vi "LabVIEW_MQTT_Toolkit_V2.vi"() -> ()   [LabVIEW 2021] (continued)
                n724 = Open/Create/Replace File(file path (use dialog)=w1674, operation (0:open)=T11."open or create") -> (refnum out=w1667:refnum<file>, error out=w1665:errorcluster)  [unwired: 4 in, 1 out]
                n725 = Write to Text File(file (use dialog)=w1667, text=w1668, error in=w1665) -> (refnum out=w1666:refnum<file>, error out=w1664:errorcluster)  [unwired: 1 in, 1 out]
                n726 = Close File(refnum=w1666, error in=w1664) -> (path=w1654:path)  [unwired: 1 out]
              }
              frame 19 {
                w1723 = T14 2 items=["User Home"=0, "User Desktop"=1, "User Documents"=2, "User Application Data"=3, "User Preferences"=4, "User Temporary"=5, "Public Documents"=6, "Public Application Data"=7, "Public Preferences"=8, "Public Cache"=13, "System Core Libraries"=9, "System Installed Libraries"=10, "Application Files"=11, "Boot Volume Root"=12] ("system directory type")
                n727 = Search and Replace String(replace all?=TRUE ("replace all? (F)"), input string=w1718, search string="/") -> (result string=w1739:string)  [unwired: 5 in, 3 out]
                n728 = Concatenate Strings(w1716, "TimeStamp;MeasureCh_Z(g);Ch_X(g);INC_Y(Deg)", "\n") -> (w1732:string)
                n729 = Concatenate Strings(w1739, "_" ("string"), "streaming.csv") -> (w1740:string)
                n730 = call <vilib>:"Get System Directory.vi"("system directory type"=w1723) -> ("system directory"=w1733:path)  [unwired: 10 in]
                n731 = Decimate 1D Array(w1756) -> (w1752:dbl[], w1751:dbl[], w1754:dbl[])
                n732 = for {
                  tunnel: [w1784] -> w1753 mode=indexing
                  tunnel: w1755 -> [w1778] mode=indexing
                  tunnel: w1752 -> [w1777] mode=indexing
                  tunnel: w1751 -> [w1776] mode=indexing
                  tunnel: w1754 -> [w1775] mode=indexing
                  tunnel: [w1777] -> w1750 mode=indexing
                  tunnel: [w1776] -> w1749 mode=indexing
                  tunnel: [w1775] -> w1748 mode=indexing
                  tunnel: w1747 -> [w1770]
                  tunnel: w1746 -> [w1769]
                  tunnel: w1745 -> [w1768] mode=indexing
                  tunnel: w1744 -> [w1767]
                  tunnel: [w1761] -> w1743
                  tunnel: [w1761] -> w1742
                  tunnel: [w1761] -> w1741
                  n733 = Join Numbers(hi=w1770, lo=w1769) -> ((hi.lo)=w1772:u32)
                  n734 = To Double Precision Float(number=w1768) -> (double precision float=w1773:dbl)
                  n735 = Number To Decimal String(number=w1778) -> (decimal integer string=w1783:string)  [unwired: 1 in]
                  n736 = Number To Fractional String(number=w1777, precision (6)=i16 3 ("width (-)")) -> (F-format string=w1785:string)  [unwired: 2 in]
                  n737 = Number To Fractional String(number=w1776, precision (6)=i16 3 ("width (-)")) -> (F-format string=w1781:string)  [unwired: 2 in]
                  n738 = Number To Fractional String(number=w1775, precision (6)=i16 3 ("width (-)")) -> (F-format string=w1779:string)  [unwired: 2 in]
                  n739 = Divide(x=w1773, y=w1767) -> (x/y=w1774:dbl)
                  n740 = To Unsigned Quad Integer(1:w1772) -> (0:w1771:u64)
                  n741 = Build Array(w1783, w1785, w1781, w1779) -> (w1784:string[])
                  n742 = call "Unix Time to Timestamp.vi"("Fractional Second"=w1774, "Unix Time (s)"=w1771) -> ("Timestamp"=w1762:timestamp)  [unwired: 8 in, 1 out]
                  n743 = Format Date/Time String(seconds (now)=w1762, UTC format=TRUE) -> (date/time string=w1763:string)  [unwired: 1 in]
                  n744 = Scan From String(format string="%<%x %H:%M:%S%3u>T", input string=w1763) -> (output 1=w1764:timestamp)  [unwired: 3 in, 3 out]
                  n745 = To Double Precision Float(number=w1764) -> (double precision float=w1761:dbl)
                }
                n746 = Build Path(base path=w1733, name or relative path="Logfile") -> (appended path=w1734:path)
                n747 = call <vilib>:"Check if File or Folder Exists.vi"("path"=w1734) -> ("file or folder exists?"=w1735:bool, "dup path"=w1736:path)  [unwired: 8 in, 1 out]
                n748 = case shown="False" w1735 {
                  tunnel: w1736 -> [w1759 w1760]
                  tunnel: [w1758 w1760] -> w1737
                  frame False {
                    n749 = Create Folder(path (use dialog)=w1759) -> (created path=w1758:path)  [unwired: 2 in, 2 out]
                  }
                  frame True {
                  }
                }
                n750 = Build Path(base path=w1737, name or relative path=w1740) -> (appended path=w1738:path)
                n751 = Open/Create/Replace File(file path (use dialog)=w1738, operation (0:open)=T11."open or create") -> (refnum out=w1731:refnum<file>, error out=w1729:errorcluster)  [unwired: 4 in, 1 out]
                n752 = Write to Text File(file (use dialog)=w1731, text=w1732, error in=w1729) -> (refnum out=w1730:refnum<file>, error out=w1728:errorcluster)  [unwired: 1 in, 1 out]
                n753 = Close File(refnum=w1730, error in=w1728) -> (path=w1717:path)  [unwired: 1 out]
              }
              frame 20 {
                w1794 = T14 2 items=["User Home"=0, "User Desktop"=1, "User Documents"=2, "User Application Data"=3, "User Preferences"=4, "User Temporary"=5, "Public Documents"=6, "Public Application Data"=7, "Public Preferences"=8, "Public Cache"=13, "System Core Libraries"=9, "System Installed Libraries"=10, "Application Files"=11, "Boot Volume Root"=12] ("system directory type")
                n754 = Decimate 1D Array(w1823) -> (w1819:dbl[], w1821:dbl[])
                n755 = Search and Replace String(replace all?=TRUE ("replace all? (F)"), input string=w1788, search string="/") -> (result string=w1810:string)  [unwired: 5 in, 3 out]
                n756 = for {
                  tunnel: [w1848] -> w1820 mode=indexing
                  tunnel: w1822 -> [w1844] mode=indexing
                  tunnel: w1819 -> [w1843] mode=indexing
                  tunnel: w1821 -> [w1842] mode=indexing
                  tunnel: [w1843] -> w1818 mode=indexing
                  tunnel: [w1842] -> w1817 mode=indexing
                  tunnel: w1816 -> [w1837]
                  tunnel: w1815 -> [w1836]
                  tunnel: w1814 -> [w1835] mode=indexing
                  tunnel: w1813 -> [w1834]
                  tunnel: [w1828] -> w1812
                  n757 = Join Numbers(hi=w1837, lo=w1836) -> ((hi.lo)=w1839:u32)
                  n758 = To Double Precision Float(number=w1835) -> (double precision float=w1840:dbl)
                  n759 = Number To Decimal String(number=w1844) -> (decimal integer string=w1847:string)  [unwired: 1 in]
                  n760 = Number To Fractional String(number=w1843, precision (6)=i16 3 ("width (-)")) -> (F-format string=w1849:string)  [unwired: 2 in]
                  n761 = Number To Fractional String(number=w1842, precision (6)=i16 3 ("width (-)")) -> (F-format string=w1845:string)  [unwired: 2 in]
                  n762 = Divide(x=w1840, y=w1834) -> (x/y=w1841:dbl)
                  n763 = Build Array(w1847, w1849, w1845) -> (w1848:string[])
                  n764 = To Unsigned Quad Integer(1:w1839) -> (0:w1838:u64)
                  n765 = call "Unix Time to Timestamp.vi"("Fractional Second"=w1841, "Unix Time (s)"=w1838) -> ("Timestamp"=w1829:timestamp)  [unwired: 8 in, 1 out]
                  n766 = Format Date/Time String(seconds (now)=w1829, UTC format=TRUE) -> (date/time string=w1830:string)  [unwired: 1 in]
                  n767 = Scan From String(format string="%<%x %H:%M:%S%3u>T", input string=w1830) -> (output 1=w1831:timestamp)  [unwired: 3 in, 3 out]
                  n768 = To Double Precision Float(number=w1831) -> (double precision float=w1828:dbl)
                }
                n769 = Concatenate Strings(w1787, "TimeStamp;MeasureCh_Y(g);INC_Y(Deg)", "\n") -> (w1803:string)
                n770 = Concatenate Strings(w1810, "_" ("string"), "streaming.csv") -> (w1811:string)
                n771 = call <vilib>:"Get System Directory.vi"("system directory type"=w1794) -> ("system directory"=w1804:path)  [unwired: 10 in]
                n772 = Build Path(base path=w1804, name or relative path="Logfile") -> (appended path=w1805:path)
                n773 = call <vilib>:"Check if File or Folder Exists.vi"("path"=w1805) -> ("file or folder exists?"=w1806:bool, "dup path"=w1807:path)  [unwired: 8 in, 1 out]
                n774 = case shown="False" w1806 {
                  tunnel: w1807 -> [w1826 w1827]
                  tunnel: [w1825 w1827] -> w1808
                  frame False {
                    n775 = Create Folder(path (use dialog)=w1826) -> (created path=w1825:path)  [unwired: 2 in, 2 out]
                  }
                  frame True {
                  }
                }
                n776 = Build Path(base path=w1808, name or relative path=w1811) -> (appended path=w1809:path)
                n777 = Open/Create/Replace File(file path (use dialog)=w1809, operation (0:open)=T11."open or create") -> (refnum out=w1802:refnum<file>, error out=w1800:errorcluster)  [unwired: 4 in, 1 out]
                n778 = Write to Text File(file (use dialog)=w1802, text=w1803, error in=w1800) -> (refnum out=w1801:refnum<file>, error out=w1799:errorcluster)  [unwired: 1 in, 1 out]
                n779 = Close File(refnum=w1801, error in=w1799) -> (path=w1789:path)  [unwired: 1 out]
              }
              frame 21 {
                w1858 = T14 2 items=["User Home"=0, "User Desktop"=1, "User Documents"=2, "User Application Data"=3, "User Preferences"=4, "User Temporary"=5, "Public Documents"=6, "Public Application Data"=7, "Public Preferences"=8, "Public Cache"=13, "System Core Libraries"=9, "System Installed Libraries"=10, "Application Files"=11, "Boot Volume Root"=12] ("system directory type")
                n780 = Search and Replace String(replace all?=TRUE ("replace all? (F)"), input string=w1853, search string="/") -> (result string=w1874:string)  [unwired: 5 in, 3 out]
                n781 = Concatenate Strings(w1851, "TimeStamp;MeasureCh_Z(g);Ch_Y(g);INC_Y(Deg)", "\n") -> (w1867:string)
                n782 = Concatenate Strings(w1874, "_" ("string"), "streaming.csv") -> (w1875:string)
                n783 = call <vilib>:"Get System Directory.vi"("system directory type"=w1858) -> ("system directory"=w1868:path)  [unwired: 10 in]
                n784 = Decimate 1D Array(w1891) -> (w1887:dbl[], w1886:dbl[], w1889:dbl[])
                n785 = for {
                  tunnel: [w1919] -> w1888 mode=indexing
                  tunnel: w1890 -> [w1913] mode=indexing
                  tunnel: w1887 -> [w1912] mode=indexing
                  tunnel: w1886 -> [w1911] mode=indexing
                  tunnel: w1889 -> [w1910] mode=indexing
                  tunnel: [w1912] -> w1885 mode=indexing
                  tunnel: [w1911] -> w1884 mode=indexing
                  tunnel: [w1910] -> w1883 mode=indexing
                  tunnel: w1882 -> [w1905]
                  tunnel: w1881 -> [w1904]
                  tunnel: w1880 -> [w1903] mode=indexing
                  tunnel: w1879 -> [w1902]
                  tunnel: [w1896] -> w1878
                  tunnel: [w1896] -> w1877
                  tunnel: [w1896] -> w1876
                  n786 = Join Numbers(hi=w1905, lo=w1904) -> ((hi.lo)=w1907:u32)
                  n787 = To Double Precision Float(number=w1903) -> (double precision float=w1908:dbl)
                  n788 = Number To Decimal String(number=w1913) -> (decimal integer string=w1918:string)  [unwired: 1 in]
                  n789 = Number To Fractional String(number=w1912, precision (6)=i16 3 ("width (-)")) -> (F-format string=w1920:string)  [unwired: 2 in]
                  n790 = Number To Fractional String(number=w1911, precision (6)=i16 3 ("width (-)")) -> (F-format string=w1916:string)  [unwired: 2 in]
                  n791 = Number To Fractional String(number=w1910, precision (6)=i16 3 ("width (-)")) -> (F-format string=w1914:string)  [unwired: 2 in]
                  n792 = Divide(x=w1908, y=w1902) -> (x/y=w1909:dbl)
                  n793 = To Unsigned Quad Integer(1:w1907) -> (0:w1906:u64)
                  n794 = Build Array(w1918, w1920, w1916, w1914) -> (w1919:string[])
                  n795 = call "Unix Time to Timestamp.vi"("Fractional Second"=w1909, "Unix Time (s)"=w1906) -> ("Timestamp"=w1897:timestamp)  [unwired: 8 in, 1 out]
                  n796 = Format Date/Time String(seconds (now)=w1897, UTC format=TRUE) -> (date/time string=w1901:string)  [unwired: 1 in]
                  n797 = Scan From String(format string="%<%x %H:%M:%S%3u>T", input string=w1901) -> (output 1=w1900:timestamp)  [unwired: 3 in, 3 out]
                  n798 = To Double Precision Float(number=w1900) -> (double precision float=w1896:dbl)
                }
                n799 = Build Path(base path=w1868, name or relative path="Logfile") -> (appended path=w1869:path)
                n800 = call <vilib>:"Check if File or Folder Exists.vi"("path"=w1869) -> ("file or folder exists?"=w1870:bool, "dup path"=w1871:path)  [unwired: 8 in, 1 out]
                n801 = case shown="False" w1870 {
                  tunnel: w1871 -> [w1894 w1895]
                  tunnel: [w1893 w1895] -> w1872
                  frame False {
                    n802 = Create Folder(path (use dialog)=w1894) -> (created path=w1893:path)  [unwired: 2 in, 2 out]
                  }
                  frame True {
                  }
                }
                n803 = Build Path(base path=w1872, name or relative path=w1875) -> (appended path=w1873:path)
                n804 = Open/Create/Replace File(file path (use dialog)=w1873, operation (0:open)=T11."open or create") -> (refnum out=w1866:refnum<file>, error out=w1864:errorcluster)  [unwired: 4 in, 1 out]
                n805 = Write to Text File(file (use dialog)=w1866, text=w1867, error in=w1864) -> (refnum out=w1865:refnum<file>, error out=w1863:errorcluster)  [unwired: 1 in, 1 out]
                n806 = Close File(refnum=w1865, error in=w1863) -> (path=w1852:path)  [unwired: 1 out]
              }
              frame 22 {
                w1929 = T14 2 items=["User Home"=0, "User Desktop"=1, "User Documents"=2, "User Application Data"=3, "User Preferences"=4, "User Temporary"=5, "Public Documents"=6, "Public Application Data"=7, "Public Preferences"=8, "Public Cache"=13, "System Core Libraries"=9, "System Installed Libraries"=10, "Application Files"=11, "Boot Volume Root"=12] ("system directory type")
                n807 = Search and Replace String(replace all?=TRUE ("replace all? (F)"), input string=w1924, search string="/") -> (result string=w1945:string)  [unwired: 5 in, 3 out]
                n808 = Concatenate Strings(w1922, "TimeStamp;MeasureCh_X(g);Ch_Y(g);INC_X(Deg)", "\n") -> (w1938:string)
                n809 = Concatenate Strings(w1945, "_" ("string"), "streaming.csv") -> (w1946:string)
                n810 = call <vilib>:"Get System Directory.vi"("system directory type"=w1929) -> ("system directory"=w1939:path)  [unwired: 10 in]
                n811 = Decimate 1D Array(w1962) -> (w1958:dbl[], w1957:dbl[], w1961:dbl[])
                n812 = for {
                  tunnel: [w1990] -> w1959 mode=indexing
                  tunnel: w1960 -> [w1984] mode=indexing
                  tunnel: w1958 -> [w1983] mode=indexing
                  tunnel: w1957 -> [w1982] mode=indexing
                  tunnel: w1961 -> [w1981] mode=indexing
                  tunnel: [w1983] -> w1956 mode=indexing
                  tunnel: [w1982] -> w1955 mode=indexing
                  tunnel: [w1981] -> w1954 mode=indexing
                  tunnel: w1953 -> [w1976]
                  tunnel: w1952 -> [w1975]
                  tunnel: w1951 -> [w1974] mode=indexing
                  tunnel: w1950 -> [w1973]
                  tunnel: [w1967] -> w1949
                  tunnel: [w1967] -> w1948
                  tunnel: [w1967] -> w1947
                  n813 = Join Numbers(hi=w1976, lo=w1975) -> ((hi.lo)=w1978:u32)
                  n814 = To Double Precision Float(number=w1974) -> (double precision float=w1979:dbl)
                  n815 = Number To Decimal String(number=w1984) -> (decimal integer string=w1989:string)  [unwired: 1 in]
                  n816 = Number To Fractional String(number=w1983, precision (6)=i16 3 ("width (-)")) -> (F-format string=w1991:string)  [unwired: 2 in]
                  n817 = Number To Fractional String(number=w1982, precision (6)=i16 3 ("width (-)")) -> (F-format string=w1987:string)  [unwired: 2 in]
                  n818 = Number To Fractional String(number=w1981, precision (6)=i16 3 ("width (-)")) -> (F-format string=w1985:string)  [unwired: 2 in]
                  n819 = Divide(x=w1979, y=w1973) -> (x/y=w1980:dbl)
                  n820 = To Unsigned Quad Integer(1:w1978) -> (0:w1977:u64)
                  n821 = Build Array(w1989, w1991, w1987, w1985) -> (w1990:string[])
                  n822 = call "Unix Time to Timestamp.vi"("Fractional Second"=w1980, "Unix Time (s)"=w1977) -> ("Timestamp"=w1968:timestamp)  [unwired: 8 in, 1 out]
                  n823 = Format Date/Time String(seconds (now)=w1968, UTC format=TRUE) -> (date/time string=w1969:string)  [unwired: 1 in]
                  n824 = Scan From String(format string="%<%x %H:%M:%S%3u>T", input string=w1969) -> (output 1=w1970:timestamp)  [unwired: 3 in, 3 out]
                  n825 = To Double Precision Float(number=w1970) -> (double precision float=w1967:dbl)
                }
                n826 = Build Path(base path=w1939, name or relative path="Logfile") -> (appended path=w1940:path)
                n827 = call <vilib>:"Check if File or Folder Exists.vi"("path"=w1940) -> ("file or folder exists?"=w1941:bool, "dup path"=w1942:path)  [unwired: 8 in, 1 out]
                n828 = case shown="False" w1941 {
                  tunnel: w1942 -> [w1965 w1966]
                  tunnel: [w1964 w1966] -> w1943
                  frame False {
                    n829 = Create Folder(path (use dialog)=w1965) -> (created path=w1964:path)  [unwired: 2 in, 2 out]
                  }
                  frame True {
                  }
                }
                n830 = Build Path(base path=w1943, name or relative path=w1946) -> (appended path=w1944:path)
                n831 = Open/Create/Replace File(file path (use dialog)=w1944, operation (0:open)=T11."open or create") -> (refnum out=w1937:refnum<file>, error out=w1935:errorcluster)  [unwired: 4 in, 1 out]
                n832 = Write to Text File(file (use dialog)=w1937, text=w1938, error in=w1935) -> (refnum out=w1936:refnum<file>, error out=w1934:errorcluster)  [unwired: 1 in, 1 out]
                n833 = Close File(refnum=w1936, error in=w1934) -> (path=w1923:path)  [unwired: 1 out]
              }
              frame 23 {
                w2000 = T14 2 items=["User Home"=0, "User Desktop"=1, "User Documents"=2, "User Application Data"=3, "User Preferences"=4, "User Temporary"=5, "Public Documents"=6, "Public Application Data"=7, "Public Preferences"=8, "Public Cache"=13, "System Core Libraries"=9, "System Installed Libraries"=10, "Application Files"=11, "Boot Volume Root"=12] ("system directory type")
                n834 = Search and Replace String(replace all?=TRUE ("replace all? (F)"), input string=w1994, search string="/") -> (result string=w2016:string)  [unwired: 5 in, 3 out]
                n835 = Concatenate Strings(w1993, "TimeStamp;MeasureCh_Z(g);Ch_X(g);Ch_Y(g);INC_Y(Deg)", "\n") -> (w2009:string)
                n836 = Concatenate Strings(w2016, "_" ("string"), "streaming.csv") -> (w2017:string)
                n837 = call <vilib>:"Get System Directory.vi"("system directory type"=w2000) -> ("system directory"=w2010:path)  [unwired: 10 in]
                n838 = Decimate 1D Array(w2033) -> (w2032:dbl[], w2031:dbl[], w2030:dbl[], w2027:dbl[])
                n839 = for {
                  tunnel: [w2063] -> w2028 mode=indexing
                  tunnel: w2029 -> [w2057] mode=indexing
                  tunnel: w2032 -> [w2055] mode=indexing
                  tunnel: w2031 -> [w2054] mode=indexing
                  tunnel: w2030 -> [w2053] mode=indexing
                  tunnel: w2027 -> [w2052] mode=indexing
                  tunnel: [w2055] -> w2026 mode=indexing
                  tunnel: [w2054] -> w2025 mode=indexing
                  tunnel: [w2053] -> w2024 mode=indexing
                  tunnel: [w2052] -> w2023 mode=indexing
                  tunnel: w2022 -> [w2047]
                  tunnel: w2021 -> [w2046]
                  tunnel: w2020 -> [w2045] mode=indexing
                  tunnel: w2019 -> [w2044]
                  tunnel: [w2038] -> w2018
                  n840 = Number To Fractional String(number=w2052, precision (6)=i16 3 ("width (-)")) -> ()  [unwired: 2 in, 1 out]
                  n841 = Join Numbers(hi=w2047, lo=w2046) -> ((hi.lo)=w2049:u32)
                  n842 = To Double Precision Float(number=w2045) -> (double precision float=w2050:dbl)
                  n843 = Number To Decimal String(number=w2057) -> (decimal integer string=w2062:string)  [unwired: 1 in]
                  n844 = Number To Fractional String(number=w2055, precision (6)=i16 3 ("width (-)")) -> (F-format string=w2064:string)  [unwired: 2 in]
                  n845 = Number To Fractional String(number=w2054, precision (6)=i16 3 ("width (-)")) -> (F-format string=w2060:string)  [unwired: 2 in]
                  n846 = Number To Fractional String(number=w2053, precision (6)=i16 3 ("width (-)")) -> (F-format string=w2058:string)  [unwired: 2 in]
                  n847 = Divide(x=w2050, y=w2044) -> (x/y=w2051:dbl)
                  n848 = To Unsigned Quad Integer(1:w2049) -> (0:w2048:u64)
                  n849 = Build Array(w2062, w2064, w2060, w2058) -> (w2063:string[])
                  n850 = call "Unix Time to Timestamp.vi"("Fractional Second"=w2051, "Unix Time (s)"=w2048) -> ("Timestamp"=w2039:timestamp)  [unwired: 8 in, 1 out]
                  n851 = Format Date/Time String(seconds (now)=w2039, UTC format=TRUE) -> (date/time string=w2040:string)  [unwired: 1 in]
                  n852 = Scan From String(format string="%<%x %H:%M:%S%3u>T", input string=w2040) -> (output 1=w2041:timestamp)  [unwired: 3 in, 3 out]
                  n853 = To Double Precision Float(number=w2041) -> (double precision float=w2038:dbl)
                }
                n854 = Build Path(base path=w2010, name or relative path="Logfile") -> (appended path=w2011:path)
                n855 = call <vilib>:"Check if File or Folder Exists.vi"("path"=w2011) -> ("file or folder exists?"=w2012:bool, "dup path"=w2013:path)  [unwired: 8 in, 1 out]
                n856 = case shown="False" w2012 {
                  tunnel: w2013 -> [w2036 w2037]
                  tunnel: [w2035 w2037] -> w2014
                  frame False {
                    n857 = Create Folder(path (use dialog)=w2036) -> (created path=w2035:path)  [unwired: 2 in, 2 out]
                  }
                  frame True {
                  }
                }
                n858 = Build Path(base path=w2014, name or relative path=w2017) -> (appended path=w2015:path)
                n859 = Open/Create/Replace File(file path (use dialog)=w2015, operation (0:open)=T11."open or create") -> (refnum out=w2008:refnum<file>, error out=w2006:errorcluster)  [unwired: 4 in, 1 out]
                n860 = Write to Text File(file (use dialog)=w2008, text=w2009, error in=w2006) -> (refnum out=w2007:refnum<file>, error out=w2005:errorcluster)  [unwired: 1 in, 1 out]
                n861 = Close File(refnum=w2007, error in=w2005) -> (path=w1995:path)  [unwired: 1 out]
              }
              frame 24 {
                w2073 = T14 2 items=["User Home"=0, "User Desktop"=1, "User Documents"=2, "User Application Data"=3, "User Preferences"=4, "User Temporary"=5, "Public Documents"=6, "Public Application Data"=7, "Public Preferences"=8, "Public Cache"=13, "System Core Libraries"=9, "System Installed Libraries"=10, "Application Files"=11, "Boot Volume Root"=12] ("system directory type")
                n862 = Decimate 1D Array(w2102) -> (w2100:dbl[], w2099:dbl[])
                n863 = Search and Replace String(replace all?=TRUE ("replace all? (F)"), input string=w2068, search string="/") -> (result string=w2089:string)  [unwired: 5 in, 3 out]
                n864 = Concatenate Strings(w2066, "TimeStamp;Measure INC_X(Deg);INC_Y(Deg)", "\n") -> (w2082:string)
                n865 = for {
                  tunnel: [w2127] -> w2098 mode=indexing
                  tunnel: w2101 -> [w2123] mode=indexing
                  tunnel: w2100 -> [w2122] mode=indexing
                  tunnel: w2099 -> [w2121] mode=indexing
                  tunnel: [w2122] -> w2097 mode=indexing
                  tunnel: [w2121] -> w2096 mode=indexing
                  tunnel: w2095 -> [w2116]
                  tunnel: w2094 -> [w2115]
                  tunnel: w2093 -> [w2114] mode=indexing
                  tunnel: w2092 -> [w2113]
                  tunnel: [w2107] -> w2091
                  n866 = Join Numbers(hi=w2116, lo=w2115) -> ((hi.lo)=w2118:u32)
                  n867 = To Double Precision Float(number=w2114) -> (double precision float=w2119:dbl)
                  n868 = Number To Decimal String(number=w2123) -> (decimal integer string=w2126:string)  [unwired: 1 in]
                  n869 = Number To Fractional String(number=w2122, precision (6)=i16 3 ("width (-)")) -> (F-format string=w2128:string)  [unwired: 2 in]
                  n870 = Number To Fractional String(number=w2121, precision (6)=i16 3 ("width (-)")) -> (F-format string=w2124:string)  [unwired: 2 in]
                  n871 = Divide(x=w2119, y=w2113) -> (x/y=w2120:dbl)
                  n872 = Build Array(w2126, w2128, w2124) -> (w2127:string[])
                  n873 = To Unsigned Quad Integer(1:w2118) -> (0:w2117:u64)
                  n874 = call "Unix Time to Timestamp.vi"("Fractional Second"=w2120, "Unix Time (s)"=w2117) -> ("Timestamp"=w2108:timestamp)  [unwired: 8 in, 1 out]
                  n875 = Format Date/Time String(seconds (now)=w2108, UTC format=TRUE) -> (date/time string=w2109:string)  [unwired: 1 in]
                  n876 = Scan From String(format string="%<%x %H:%M:%S%3u>T", input string=w2109) -> (output 1=w2110:timestamp)  [unwired: 3 in, 3 out]
                  n877 = To Double Precision Float(number=w2110) -> (double precision float=w2107:dbl)
                }
                n878 = Concatenate Strings(w2089, "_" ("string"), "streaming.csv") -> (w2090:string)
                n879 = call <vilib>:"Get System Directory.vi"("system directory type"=w2073) -> ("system directory"=w2083:path)  [unwired: 10 in]
                n880 = Build Path(base path=w2083, name or relative path="Logfile") -> (appended path=w2084:path)
                n881 = call <vilib>:"Check if File or Folder Exists.vi"("path"=w2084) -> ("file or folder exists?"=w2085:bool, "dup path"=w2086:path)  [unwired: 8 in, 1 out]
                n882 = case shown="False" w2085 {
                  tunnel: w2086 -> [w2105 w2106]
                  tunnel: [w2104 w2106] -> w2087
                  frame False {
                    n883 = Create Folder(path (use dialog)=w2105) -> (created path=w2104:path)  [unwired: 2 in, 2 out]
                  }
                  frame True {
                  }
                }
                n884 = Build Path(base path=w2087, name or relative path=w2090) -> (appended path=w2088:path)
                n885 = Open/Create/Replace File(file path (use dialog)=w2088, operation (0:open)=T11."open or create") -> (refnum out=w2081:refnum<file>, error out=w2079:errorcluster)  [unwired: 4 in, 1 out]
                n886 = Write to Text File(file (use dialog)=w2081, text=w2082, error in=w2079) -> (refnum out=w2080:refnum<file>, error out=w2078:errorcluster)  [unwired: 1 in, 1 out]
                n887 = Close File(refnum=w2080, error in=w2078) -> (path=w2067:path)  [unwired: 1 out]
              }
              frame 25 {
                w2137 = T14 2 items=["User Home"=0, "User Desktop"=1, "User Documents"=2, "User Application Data"=3, "User Preferences"=4, "User Temporary"=5, "Public Documents"=6, "Public Application Data"=7, "Public Preferences"=8, "Public Cache"=13, "System Core Libraries"=9, "System Installed Libraries"=10, "Application Files"=11, "Boot Volume Root"=12] ("system directory type")
                n888 = Search and Replace String(replace all?=TRUE ("replace all? (F)"), input string=w2132, search string="/") -> (result string=w2153:string)  [unwired: 5 in, 3 out]
                n889 = Concatenate Strings(w2130, "TimeStamp;Measure Ch_Z(g);INC_X(Deg);INC_Y(Deg)", "\n") -> (w2146:string)
                n890 = Concatenate Strings(w2153, "_" ("string"), "streaming.csv") -> (w2154:string)
                n891 = call <vilib>:"Get System Directory.vi"("system directory type"=w2137) -> ("system directory"=w2147:path)  [unwired: 10 in]
                n892 = Decimate 1D Array(w2168) -> (w2163:dbl[], w2166:dbl[], w2165:dbl[])
                n893 = for {
                  tunnel: [w2196] -> w2164 mode=indexing
                  tunnel: w2167 -> [w2190] mode=indexing
                  tunnel: w2163 -> [w2189] mode=indexing
                  tunnel: w2166 -> [w2188] mode=indexing
                  tunnel: w2165 -> [w2187] mode=indexing
                  tunnel: [w2189] -> w2162 mode=indexing
                  tunnel: [w2188] -> w2161 mode=indexing
                  tunnel: [w2187] -> w2160 mode=indexing
                  tunnel: w2159 -> [w2182]
                  tunnel: w2158 -> [w2181]
                  tunnel: w2157 -> [w2180] mode=indexing
                  tunnel: w2156 -> [w2179]
                  tunnel: [w2173] -> w2155
                  n894 = Join Numbers(hi=w2182, lo=w2181) -> ((hi.lo)=w2184:u32)
                  n895 = To Double Precision Float(number=w2180) -> (double precision float=w2185:dbl)
                  n896 = Number To Decimal String(number=w2190) -> (decimal integer string=w2195:string)  [unwired: 1 in]
                  n897 = Number To Fractional String(number=w2189, precision (6)=i16 3 ("width (-)")) -> (F-format string=w2197:string)  [unwired: 2 in]
                  n898 = Number To Fractional String(number=w2188, precision (6)=i16 3 ("width (-)")) -> (F-format string=w2193:string)  [unwired: 2 in]
                  n899 = Number To Fractional String(number=w2187, precision (6)=i16 3 ("width (-)")) -> (F-format string=w2191:string)  [unwired: 2 in]
                  n900 = Divide(x=w2185, y=w2179) -> (x/y=w2186:dbl)
                  n901 = To Unsigned Quad Integer(1:w2184) -> (0:w2183:u64)
                  n902 = Build Array(w2195, w2197, w2193, w2191) -> (w2196:string[])
                  n903 = call "Unix Time to Timestamp.vi"("Fractional Second"=w2186, "Unix Time (s)"=w2183) -> ("Timestamp"=w2174:timestamp)  [unwired: 8 in, 1 out]
                  n904 = Format Date/Time String(seconds (now)=w2174, UTC format=TRUE) -> (date/time string=w2175:string)  [unwired: 1 in]
                  n905 = Scan From String(format string="%<%x %H:%M:%S%3u>T", input string=w2175) -> (output 1=w2176:timestamp)  [unwired: 3 in, 3 out]
                  n906 = To Double Precision Float(number=w2176) -> (double precision float=w2173:dbl)
                }
                n907 = Build Path(base path=w2147, name or relative path="Logfile") -> (appended path=w2148:path)
                n908 = call <vilib>:"Check if File or Folder Exists.vi"("path"=w2148) -> ("file or folder exists?"=w2149:bool, "dup path"=w2150:path)  [unwired: 8 in, 1 out]
                n909 = case shown="False" w2149 {
                  tunnel: w2150 -> [w2171 w2172]
                  tunnel: [w2170 w2172] -> w2151
                  frame False {
                    n910 = Create Folder(path (use dialog)=w2171) -> (created path=w2170:path)  [unwired: 2 in, 2 out]
                  }
                  frame True {
                  }
                }
                n911 = Build Path(base path=w2151, name or relative path=w2154) -> (appended path=w2152:path)
                n912 = Open/Create/Replace File(file path (use dialog)=w2152, operation (0:open)=T11."open or create") -> (refnum out=w2145:refnum<file>, error out=w2143:errorcluster)  [unwired: 4 in, 1 out]
                n913 = Write to Text File(file (use dialog)=w2145, text=w2146, error in=w2143) -> (refnum out=w2144:refnum<file>, error out=w2142:errorcluster)  [unwired: 1 in, 1 out]
                n914 = Close File(refnum=w2144, error in=w2142) -> (path=w2131:path)  [unwired: 1 out]
              }
              frame 26 {
                w2206 = T14 2 items=["User Home"=0, "User Desktop"=1, "User Documents"=2, "User Application Data"=3, "User Preferences"=4, "User Temporary"=5, "Public Documents"=6, "Public Application Data"=7, "Public Preferences"=8, "Public Cache"=13, "System Core Libraries"=9, "System Installed Libraries"=10, "Application Files"=11, "Boot Volume Root"=12] ("system directory type")
                n915 = Search and Replace String(replace all?=TRUE ("replace all? (F)"), input string=w2201, search string="/") -> (result string=w2222:string)  [unwired: 5 in, 3 out]
                n916 = Concatenate Strings(w2199, "TimeStamp;Measure Ch_X(g);INC_X(Deg);INC_Y(Deg)", "\n") -> (w2215:string)
                n917 = Concatenate Strings(w2222, "_" ("string"), "streaming.csv") -> (w2223:string)
                n918 = call <vilib>:"Get System Directory.vi"("system directory type"=w2206) -> ("system directory"=w2216:path)  [unwired: 10 in]
                n919 = Decimate 1D Array(w2237) -> (w2232:dbl[], w2236:dbl[], w2235:dbl[])
                n920 = for {
                  tunnel: [w2265] -> w2233 mode=indexing
                  tunnel: w2234 -> [w2259] mode=indexing
                  tunnel: w2232 -> [w2258] mode=indexing
                  tunnel: w2236 -> [w2257] mode=indexing
                  tunnel: w2235 -> [w2256] mode=indexing
                  tunnel: [w2258] -> w2231 mode=indexing
                  tunnel: [w2257] -> w2230 mode=indexing
                  tunnel: [w2256] -> w2229 mode=indexing
                  tunnel: w2228 -> [w2251]
                  tunnel: w2227 -> [w2250]
                  tunnel: w2226 -> [w2249] mode=indexing
                  tunnel: w2225 -> [w2248]
                  tunnel: [w2242] -> w2224
                  n921 = Join Numbers(hi=w2251, lo=w2250) -> ((hi.lo)=w2253:u32)
                  n922 = To Double Precision Float(number=w2249) -> (double precision float=w2254:dbl)
                  n923 = Number To Decimal String(number=w2259) -> (decimal integer string=w2264:string)  [unwired: 1 in]
                  n924 = Number To Fractional String(number=w2258, precision (6)=i16 3 ("width (-)")) -> (F-format string=w2266:string)  [unwired: 2 in]
                  n925 = Number To Fractional String(number=w2257, precision (6)=i16 3 ("width (-)")) -> (F-format string=w2262:string)  [unwired: 2 in]
                  n926 = Number To Fractional String(number=w2256, precision (6)=i16 3 ("width (-)")) -> (F-format string=w2260:string)  [unwired: 2 in]
                  n927 = Divide(x=w2254, y=w2248) -> (x/y=w2255:dbl)
                  n928 = To Unsigned Quad Integer(1:w2253) -> (0:w2252:u64)
                  n929 = Build Array(w2264, w2266, w2262, w2260) -> (w2265:string[])
                  n930 = call "Unix Time to Timestamp.vi"("Fractional Second"=w2255, "Unix Time (s)"=w2252) -> ("Timestamp"=w2243:timestamp)  [unwired: 8 in, 1 out]
                  n931 = Format Date/Time String(seconds (now)=w2243, UTC format=TRUE) -> (date/time string=w2244:string)  [unwired: 1 in]
                  n932 = Scan From String(format string="%<%x %H:%M:%S%3u>T", input string=w2244) -> (output 1=w2245:timestamp)  [unwired: 3 in, 3 out]
                  n933 = To Double Precision Float(number=w2245) -> (double precision float=w2242:dbl)
                }
                n934 = Build Path(base path=w2216, name or relative path="Logfile") -> (appended path=w2217:path)
                n935 = call <vilib>:"Check if File or Folder Exists.vi"("path"=w2217) -> ("file or folder exists?"=w2218:bool, "dup path"=w2219:path)  [unwired: 8 in, 1 out]
                n936 = case shown="False" w2218 {
                  tunnel: w2219 -> [w2240 w2241]
                  tunnel: [w2239 w2241] -> w2220
                  frame False {
                    n937 = Create Folder(path (use dialog)=w2240) -> (created path=w2239:path)  [unwired: 2 in, 2 out]
                  }
                  frame True {
                  }
                }
                n938 = Build Path(base path=w2220, name or relative path=w2223) -> (appended path=w2221:path)
                n939 = Open/Create/Replace File(file path (use dialog)=w2221, operation (0:open)=T11."open or create") -> (refnum out=w2214:refnum<file>, error out=w2212:errorcluster)  [unwired: 4 in, 1 out]
                n940 = Write to Text File(file (use dialog)=w2214, text=w2215, error in=w2212) -> (refnum out=w2213:refnum<file>, error out=w2211:errorcluster)  [unwired: 1 in, 1 out]
                n941 = Close File(refnum=w2213, error in=w2211) -> (path=w2200:path)  [unwired: 1 out]
              }
              frame 27 {
                w2275 = T14 2 items=["User Home"=0, "User Desktop"=1, "User Documents"=2, "User Application Data"=3, "User Preferences"=4, "User Temporary"=5, "Public Documents"=6, "Public Application Data"=7, "Public Preferences"=8, "Public Cache"=13, "System Core Libraries"=9, "System Installed Libraries"=10, "Application Files"=11, "Boot Volume Root"=12] ("system directory type")
                n942 = Search and Replace String(replace all?=TRUE ("replace all? (F)"), input string=w2270, search string="/") -> (result string=w2291:string)  [unwired: 5 in, 3 out]
                n943 = Concatenate Strings(w2268, "TimeStamp;Measure Ch_Z(g);Ch_X(g);INC_X(Deg);INC_Y(Deg)", "\n") -> (w2284:string)
                n944 = Concatenate Strings(w2291, "_" ("string"), "streaming.csv") -> (w2292:string)
                n945 = call <vilib>:"Get System Directory.vi"("system directory type"=w2275) -> ("system directory"=w2285:path)  [unwired: 10 in]
                n946 = Decimate 1D Array(w2308) -> (w2306:dbl[], w2305:dbl[], w2303:dbl[], w2302:dbl[])
                n947 = for {
                  tunnel: [w2339] -> w2307 mode=indexing
                  tunnel: w2304 -> [w2333] mode=indexing
                  tunnel: w2306 -> [w2330] mode=indexing
                  tunnel: w2305 -> [w2329] mode=indexing
                  tunnel: w2303 -> [w2328] mode=indexing
                  tunnel: w2302 -> [w2327] mode=indexing
                  tunnel: [w2330] -> w2301 mode=indexing
                  tunnel: [w2329] -> w2300 mode=indexing
                  tunnel: [w2328] -> w2299 mode=indexing
                  tunnel: [w2327] -> w2298 mode=indexing
                  tunnel: w2297 -> [w2322]
                  tunnel: w2296 -> [w2321]
                  tunnel: w2295 -> [w2320] mode=indexing
                  tunnel: w2294 -> [w2319]
                  tunnel: [w2313] -> w2293
                  n948 = Join Numbers(hi=w2322, lo=w2321) -> ((hi.lo)=w2324:u32)
                  n949 = To Double Precision Float(number=w2320) -> (double precision float=w2325:dbl)
                  n950 = Number To Decimal String(number=w2333) -> (decimal integer string=w2338:string)  [unwired: 1 in]
                  n951 = Number To Fractional String(number=w2330, precision (6)=i16 3 ("width (-)")) -> (F-format string=w2340:string)  [unwired: 2 in]
                  n952 = Number To Fractional String(number=w2329, precision (6)=i16 3 ("width (-)")) -> (F-format string=w2336:string)  [unwired: 2 in]
                  n953 = Number To Fractional String(number=w2328, precision (6)=i16 3 ("width (-)")) -> (F-format string=w2334:string)  [unwired: 2 in]
                  n954 = Number To Fractional String(number=w2327, precision (6)=i16 3 ("width (-)")) -> (F-format string=w2331:string)  [unwired: 2 in]
                  n955 = Divide(x=w2325, y=w2319) -> (x/y=w2326:dbl)
                  n956 = To Unsigned Quad Integer(1:w2324) -> (0:w2323:u64)
                  n957 = Build Array(w2338, w2340, w2336, w2334, w2331) -> (w2339:string[])
                  n958 = call "Unix Time to Timestamp.vi"("Fractional Second"=w2326, "Unix Time (s)"=w2323) -> ("Timestamp"=w2314:timestamp)  [unwired: 8 in, 1 out]
                  n959 = Format Date/Time String(seconds (now)=w2314, UTC format=TRUE) -> (date/time string=w2318:string)  [unwired: 1 in]
                  n960 = Scan From String(format string="%<%x %H:%M:%S%3u>T", input string=w2318) -> (output 1=w2317:timestamp)  [unwired: 3 in, 3 out]
                  n961 = To Double Precision Float(number=w2317) -> (double precision float=w2313:dbl)
                }
                n962 = Build Path(base path=w2285, name or relative path="Logfile") -> (appended path=w2286:path)
                n963 = call <vilib>:"Check if File or Folder Exists.vi"("path"=w2286) -> ("file or folder exists?"=w2287:bool, "dup path"=w2288:path)  [unwired: 8 in, 1 out]
                n964 = case shown="False" w2287 {
                  tunnel: w2288 -> [w2311 w2312]
                  tunnel: [w2310 w2312] -> w2289
                  frame False {
                    n965 = Create Folder(path (use dialog)=w2311) -> (created path=w2310:path)  [unwired: 2 in, 2 out]
                  }
                  frame True {
                  }
                }
                n966 = Build Path(base path=w2289, name or relative path=w2292) -> (appended path=w2290:path)
                n967 = Open/Create/Replace File(file path (use dialog)=w2290, operation (0:open)=T11."open or create") -> (refnum out=w2283:refnum<file>, error out=w2281:errorcluster)  [unwired: 4 in, 1 out]
                n968 = Write to Text File(file (use dialog)=w2283, text=w2284, error in=w2281) -> (refnum out=w2282:refnum<file>, error out=w2280:errorcluster)  [unwired: 1 in, 1 out]
                n969 = Close File(refnum=w2282, error in=w2280) -> (path=w2269:path)  [unwired: 1 out]
              }
              frame 28 {
                w2349 = T14 2 items=["User Home"=0, "User Desktop"=1, "User Documents"=2, "User Application Data"=3, "User Preferences"=4, "User Temporary"=5, "Public Documents"=6, "Public Application Data"=7, "Public Preferences"=8, "Public Cache"=13, "System Core Libraries"=9, "System Installed Libraries"=10, "Application Files"=11, "Boot Volume Root"=12] ("system directory type")
                n970 = Search and Replace String(replace all?=TRUE ("replace all? (F)"), input string=w2344, search string="/") -> (result string=w2365:string)  [unwired: 5 in, 3 out]
                n971 = Concatenate Strings(w2342, "TimeStamp;Measure Ch_Y(g);INC_X(Deg);INC_Y(Deg)", "\n") -> (w2358:string)
                n972 = Concatenate Strings(w2365, "_" ("string"), "streaming.csv") -> (w2366:string)
                n973 = call <vilib>:"Get System Directory.vi"("system directory type"=w2349) -> ("system directory"=w2359:path)  [unwired: 10 in]
                n974 = Decimate 1D Array(w2380) -> (w2378:dbl[], w2377:dbl[], w2376:dbl[])
                n975 = for {
                  tunnel: [w2408] -> w2375 mode=indexing
                  tunnel: w2379 -> [w2402] mode=indexing
                  tunnel: w2378 -> [w2401] mode=indexing
                  tunnel: w2377 -> [w2400] mode=indexing
                  tunnel: w2376 -> [w2399] mode=indexing
                  tunnel: [w2401] -> w2374 mode=indexing
                  tunnel: [w2400] -> w2373 mode=indexing
                  tunnel: [w2399] -> w2372 mode=indexing
                  tunnel: w2371 -> [w2394]
                  tunnel: w2370 -> [w2393]
                  tunnel: w2369 -> [w2392] mode=indexing
                  tunnel: w2368 -> [w2391]
                  tunnel: [w2385] -> w2367
                  n976 = Join Numbers(hi=w2394, lo=w2393) -> ((hi.lo)=w2396:u32)
                  n977 = To Double Precision Float(number=w2392) -> (double precision float=w2397:dbl)
                  n978 = Number To Decimal String(number=w2402) -> (decimal integer string=w2407:string)  [unwired: 1 in]
                  n979 = Number To Fractional String(number=w2401, precision (6)=i16 3 ("width (-)")) -> (F-format string=w2409:string)  [unwired: 2 in]
                  n980 = Number To Fractional String(number=w2400, precision (6)=i16 3 ("width (-)")) -> (F-format string=w2405:string)  [unwired: 2 in]
                  n981 = Number To Fractional String(number=w2399, precision (6)=i16 3 ("width (-)")) -> (F-format string=w2403:string)  [unwired: 2 in]
                  n982 = Divide(x=w2397, y=w2391) -> (x/y=w2398:dbl)
                  n983 = To Unsigned Quad Integer(1:w2396) -> (0:w2395:u64)
                  n984 = Build Array(w2407, w2409, w2405, w2403) -> (w2408:string[])
                  n985 = call "Unix Time to Timestamp.vi"("Fractional Second"=w2398, "Unix Time (s)"=w2395) -> ("Timestamp"=w2386:timestamp)  [unwired: 8 in, 1 out]
                  n986 = Format Date/Time String(seconds (now)=w2386, UTC format=TRUE) -> (date/time string=w2387:string)  [unwired: 1 in]
                  n987 = Scan From String(format string="%<%x %H:%M:%S%3u>T", input string=w2387) -> (output 1=w2388:timestamp)  [unwired: 3 in, 3 out]
                  n988 = To Double Precision Float(number=w2388) -> (double precision float=w2385:dbl)
                }
                n989 = Build Path(base path=w2359, name or relative path="Logfile") -> (appended path=w2360:path)
                n990 = call <vilib>:"Check if File or Folder Exists.vi"("path"=w2360) -> ("file or folder exists?"=w2361:bool, "dup path"=w2362:path)  [unwired: 8 in, 1 out]
                n991 = case shown="False" w2361 {
                  tunnel: w2362 -> [w2383 w2384]
                  tunnel: [w2382 w2384] -> w2363
                  frame False {
                    n992 = Create Folder(path (use dialog)=w2383) -> (created path=w2382:path)  [unwired: 2 in, 2 out]
                  }
                  frame True {
                  }
                }
                n993 = Build Path(base path=w2363, name or relative path=w2366) -> (appended path=w2364:path)
                n994 = Open/Create/Replace File(file path (use dialog)=w2364, operation (0:open)=T11."open or create") -> (refnum out=w2357:refnum<file>, error out=w2355:errorcluster)  [unwired: 4 in, 1 out]
                n995 = Write to Text File(file (use dialog)=w2357, text=w2358, error in=w2355) -> (refnum out=w2356:refnum<file>, error out=w2354:errorcluster)  [unwired: 1 in, 1 out]
                n996 = Close File(refnum=w2356, error in=w2354) -> (path=w2343:path)  [unwired: 1 out]
              }
              frame 29 {
                w2418 = T14 2 items=["User Home"=0, "User Desktop"=1, "User Documents"=2, "User Application Data"=3, "User Preferences"=4, "User Temporary"=5, "Public Documents"=6, "Public Application Data"=7, "Public Preferences"=8, "Public Cache"=13, "System Core Libraries"=9, "System Installed Libraries"=10, "Application Files"=11, "Boot Volume Root"=12] ("system directory type")
                n997 = Search and Replace String(replace all?=TRUE ("replace all? (F)"), input string=w2413, search string="/") -> (result string=w2434:string)  [unwired: 5 in, 3 out]
                n998 = Concatenate Strings(w2411, "TimeStamp;Measure Ch_Z(g);Ch_Y(g);INC_X(Deg);INC_Y(Deg)", "\n") -> (w2427:string)
                n999 = Concatenate Strings(w2434, "_" ("string"), "streaming.csv") -> (w2435:string)
                n1000 = call <vilib>:"Get System Directory.vi"("system directory type"=w2418) -> ("system directory"=w2428:path)  [unwired: 10 in]
                n1001 = Decimate 1D Array(w2451) -> (w2445:dbl[], w2449:dbl[], w2446:dbl[], w2447:dbl[])
                n1002 = for {
                  tunnel: [w2482] -> w2448 mode=indexing
                  tunnel: w2450 -> [w2476] mode=indexing
                  tunnel: w2445 -> [w2473] mode=indexing
                  tunnel: w2449 -> [w2472] mode=indexing
                  tunnel: w2446 -> [w2471] mode=indexing
                  tunnel: w2447 -> [w2470] mode=indexing
                  tunnel: [w2473] -> w2444 mode=indexing
                  tunnel: [w2472] -> w2443 mode=indexing
                  tunnel: [w2471] -> w2442 mode=indexing
                  tunnel: [w2470] -> w2441 mode=indexing
                  tunnel: w2440 -> [w2465]
                  tunnel: w2439 -> [w2464]
                  tunnel: w2438 -> [w2463] mode=indexing
                  tunnel: w2437 -> [w2462]
                  tunnel: [w2456] -> w2436
                  n1003 = Join Numbers(hi=w2465, lo=w2464) -> ((hi.lo)=w2467:u32)
                  n1004 = To Double Precision Float(number=w2463) -> (double precision float=w2468:dbl)
                  n1005 = Number To Decimal String(number=w2476) -> (decimal integer string=w2481:string)  [unwired: 1 in]
                  n1006 = Number To Fractional String(number=w2473, precision (6)=i16 3 ("width (-)")) -> (F-format string=w2483:string)  [unwired: 2 in]
                  n1007 = Number To Fractional String(number=w2472, precision (6)=i16 3 ("width (-)")) -> (F-format string=w2479:string)  [unwired: 2 in]
                  n1008 = Number To Fractional String(number=w2471, precision (6)=i16 3 ("width (-)")) -> (F-format string=w2477:string)  [unwired: 2 in]
                  n1009 = Number To Fractional String(number=w2470, precision (6)=i16 3 ("width (-)")) -> (F-format string=w2474:string)  [unwired: 2 in]
                  n1010 = Divide(x=w2468, y=w2462) -> (x/y=w2469:dbl)
                  n1011 = To Unsigned Quad Integer(1:w2467) -> (0:w2466:u64)
                  n1012 = Build Array(w2481, w2483, w2479, w2477, w2474) -> (w2482:string[])
                  n1013 = call "Unix Time to Timestamp.vi"("Fractional Second"=w2469, "Unix Time (s)"=w2466) -> ("Timestamp"=w2457:timestamp)  [unwired: 8 in, 1 out]
                  n1014 = Format Date/Time String(seconds (now)=w2457, UTC format=TRUE) -> (date/time string=w2458:string)  [unwired: 1 in]
                  n1015 = Scan From String(format string="%<%x %H:%M:%S%3u>T", input string=w2458) -> (output 1=w2459:timestamp)  [unwired: 3 in, 3 out]
                  n1016 = To Double Precision Float(number=w2459) -> (double precision float=w2456:dbl)
                }
                n1017 = Build Path(base path=w2428, name or relative path="Logfile") -> (appended path=w2429:path)
                n1018 = call <vilib>:"Check if File or Folder Exists.vi"("path"=w2429) -> ("file or folder exists?"=w2430:bool, "dup path"=w2431:path)  [unwired: 8 in, 1 out]
                n1019 = case shown="False" w2430 {
                  tunnel: w2431 -> [w2454 w2455]
                  tunnel: [w2453 w2455] -> w2432
                  frame False {
                    n1020 = Create Folder(path (use dialog)=w2454) -> (created path=w2453:path)  [unwired: 2 in, 2 out]
                  }
                  frame True {
                  }
                }
                n1021 = Build Path(base path=w2432, name or relative path=w2435) -> (appended path=w2433:path)
                n1022 = Open/Create/Replace File(file path (use dialog)=w2433, operation (0:open)=T11."open or create") -> (refnum out=w2426:refnum<file>, error out=w2424:errorcluster)  [unwired: 4 in, 1 out]
                n1023 = Write to Text File(file (use dialog)=w2426, text=w2427, error in=w2424) -> (refnum out=w2425:refnum<file>, error out=w2423:errorcluster)  [unwired: 1 in, 1 out]
                n1024 = Close File(refnum=w2425, error in=w2423) -> (path=w2412:path)  [unwired: 1 out]
              }
              frame 30 {
                w2492 = T14 2 items=["User Home"=0, "User Desktop"=1, "User Documents"=2, "User Application Data"=3, "User Preferences"=4, "User Temporary"=5, "Public Documents"=6, "Public Application Data"=7, "Public Preferences"=8, "Public Cache"=13, "System Core Libraries"=9, "System Installed Libraries"=10, "Application Files"=11, "Boot Volume Root"=12] ("system directory type")
                n1025 = Search and Replace String(replace all?=TRUE ("replace all? (F)"), input string=w2487, search string="/") -> (result string=w2508:string)  [unwired: 5 in, 3 out]
                n1026 = Concatenate Strings(w2485, "TimeStamp;Measure Ch_X(g);Ch_Y(g);INC_X(Deg);INC_Y(Deg)", "\n") -> (w2501:string)
                n1027 = Concatenate Strings(w2508, "_" ("string"), "streaming.csv") -> (w2509:string)
                n1028 = call <vilib>:"Get System Directory.vi"("system directory type"=w2492) -> ("system directory"=w2502:path)  [unwired: 10 in]
                n1029 = Decimate 1D Array(w2525) -> (w2524:dbl[], w2522:dbl[], w2520:dbl[], w2521:dbl[])
                n1030 = for {
                  tunnel: [w2556] -> w2519 mode=indexing
                  tunnel: w2523 -> [w2550] mode=indexing
                  tunnel: w2524 -> [w2547] mode=indexing
                  tunnel: w2522 -> [w2546] mode=indexing
                  tunnel: w2520 -> [w2545] mode=indexing
                  tunnel: w2521 -> [w2544] mode=indexing
                  tunnel: [w2547] -> w2518 mode=indexing
                  tunnel: [w2546] -> w2517 mode=indexing
                  tunnel: [w2545] -> w2516 mode=indexing
                  tunnel: [w2544] -> w2515 mode=indexing
                  tunnel: w2514 -> [w2539]
                  tunnel: w2513 -> [w2538]
                  tunnel: w2512 -> [w2537] mode=indexing
                  tunnel: w2511 -> [w2536]
                  tunnel: [w2530] -> w2510
                  n1031 = Join Numbers(hi=w2539, lo=w2538) -> ((hi.lo)=w2541:u32)
                  n1032 = To Double Precision Float(number=w2537) -> (double precision float=w2542:dbl)
                  n1033 = Number To Decimal String(number=w2550) -> (decimal integer string=w2555:string)  [unwired: 1 in]
                  n1034 = Number To Fractional String(number=w2547, precision (6)=i16 3 ("width (-)")) -> (F-format string=w2557:string)  [unwired: 2 in]
                  n1035 = Number To Fractional String(number=w2546, precision (6)=i16 3 ("width (-)")) -> (F-format string=w2553:string)  [unwired: 2 in]
                  n1036 = Number To Fractional String(number=w2545, precision (6)=i16 3 ("width (-)")) -> (F-format string=w2551:string)  [unwired: 2 in]
                  n1037 = Number To Fractional String(number=w2544, precision (6)=i16 3 ("width (-)")) -> (F-format string=w2548:string)  [unwired: 2 in]
                  n1038 = Divide(x=w2542, y=w2536) -> (x/y=w2543:dbl)
                  n1039 = To Unsigned Quad Integer(1:w2541) -> (0:w2540:u64)
                  n1040 = Build Array(w2555, w2557, w2553, w2551, w2548) -> (w2556:string[])
                  n1041 = call "Unix Time to Timestamp.vi"("Fractional Second"=w2543, "Unix Time (s)"=w2540) -> ("Timestamp"=w2531:timestamp)  [unwired: 8 in, 1 out]
                  n1042 = Format Date/Time String(seconds (now)=w2531, UTC format=TRUE) -> (date/time string=w2532:string)  [unwired: 1 in]
                  n1043 = Scan From String(format string="%<%x %H:%M:%S%3u>T", input string=w2532) -> (output 1=w2533:timestamp)  [unwired: 3 in, 3 out]
                  n1044 = To Double Precision Float(number=w2533) -> (double precision float=w2530:dbl)
                }
                n1045 = Build Path(base path=w2502, name or relative path="Logfile") -> (appended path=w2503:path)
                n1046 = call <vilib>:"Check if File or Folder Exists.vi"("path"=w2503) -> ("file or folder exists?"=w2504:bool, "dup path"=w2505:path)  [unwired: 8 in, 1 out]
                n1047 = case shown="False" w2504 {
                  tunnel: w2505 -> [w2528 w2529]
                  tunnel: [w2527 w2529] -> w2506
                  frame False {
                    n1048 = Create Folder(path (use dialog)=w2528) -> (created path=w2527:path)  [unwired: 2 in, 2 out]
                  }
                  frame True {
                  }
                }
                n1049 = Build Path(base path=w2506, name or relative path=w2509) -> (appended path=w2507:path)
                n1050 = Open/Create/Replace File(file path (use dialog)=w2507, operation (0:open)=T11."open or create") -> (refnum out=w2500:refnum<file>, error out=w2498:errorcluster)  [unwired: 4 in, 1 out]
                n1051 = Write to Text File(file (use dialog)=w2500, text=w2501, error in=w2498) -> (refnum out=w2499:refnum<file>, error out=w2497:errorcluster)  [unwired: 1 in, 1 out]
                n1052 = Close File(refnum=w2499, error in=w2497) -> (path=w2486:path)  [unwired: 1 out]
              }
              frame 31 {
                w2566 = T14 2 items=["User Home"=0, "User Desktop"=1, "User Documents"=2, "User Application Data"=3, "User Preferences"=4, "User Temporary"=5, "Public Documents"=6, "Public Application Data"=7, "Public Preferences"=8, "Public Cache"=13, "System Core Libraries"=9, "System Installed Libraries"=10, "Application Files"=11, "Boot Volume Root"=12] ("system directory type")
                n1053 = Search and Replace String(replace all?=TRUE ("replace all? (F)"), input string=w2561, search string="/") -> (result string=w2582:string)  [unwired: 5 in, 3 out]
                n1054 = Concatenate Strings(w2559, "TimeStamp;Measure Ch_Z(g);Ch_X(g);Ch_Y(g);INC_X(Deg);INC_Y(Deg)", "\n") -> (w2575:string)
                n1055 = Concatenate Strings(w2582, "_" ("string"), "streaming.csv") -> (w2583:string)
                n1056 = call <vilib>:"Get System Directory.vi"("system directory type"=w2566) -> ("system directory"=w2576:path)  [unwired: 10 in]
                n1057 = Decimate 1D Array(w2601) -> (w2600:dbl[], w2599:dbl[], w2598:dbl[], w2597:dbl[], w2595:dbl[])
                n1058 = for {
                  tunnel: [w2635] -> w2594 mode=indexing
                  tunnel: w2596 -> [w2629] mode=indexing
                  tunnel: w2600 -> [w2624] mode=indexing
                  tunnel: w2599 -> [w2623] mode=indexing
                  tunnel: w2598 -> [w2622] mode=indexing
                  tunnel: w2597 -> [w2621] mode=indexing
                  tunnel: w2595 -> [w2620] mode=indexing
                  tunnel: [w2624] -> w2593 mode=indexing
                  tunnel: [w2623] -> w2592 mode=indexing
                  tunnel: [w2622] -> w2591 mode=indexing
                  tunnel: [w2621] -> w2590 mode=indexing
                  tunnel: [w2620] -> w2589 mode=indexing
                  tunnel: w2588 -> [w2615]
                  tunnel: w2587 -> [w2614]
                  tunnel: w2586 -> [w2613] mode=indexing
                  tunnel: w2585 -> [w2612]
                  tunnel: [w2606] -> w2584
                  n1059 = Join Numbers(hi=w2615, lo=w2614) -> ((hi.lo)=w2617:u32)
                  n1060 = To Double Precision Float(number=w2613) -> (double precision float=w2618:dbl)
                  n1061 = Number To Decimal String(number=w2629) -> (decimal integer string=w2634:string)  [unwired: 1 in]
                  n1062 = Number To Fractional String(number=w2624, precision (6)=i16 3 ("width (-)")) -> (F-format string=w2636:string)  [unwired: 2 in]
                  n1063 = Number To Fractional String(number=w2623, precision (6)=i16 3 ("width (-)")) -> (F-format string=w2632:string)  [unwired: 2 in]
                  n1064 = Number To Fractional String(number=w2622, precision (6)=i16 3 ("width (-)")) -> (F-format string=w2630:string)  [unwired: 2 in]
                  n1065 = Number To Fractional String(number=w2621, precision (6)=i16 3 ("width (-)")) -> (F-format string=w2627:string)  [unwired: 2 in]
                  n1066 = Number To Fractional String(number=w2620, precision (6)=i16 3 ("width (-)")) -> (F-format string=w2625:string)  [unwired: 2 in]
                  n1067 = Divide(x=w2618, y=w2612) -> (x/y=w2619:dbl)
                  n1068 = To Unsigned Quad Integer(1:w2617) -> (0:w2616:u64)
                  n1069 = Build Array(w2634, w2636, w2632, w2630, w2627, w2625) -> (w2635:string[])
                  n1070 = call "Unix Time to Timestamp.vi"("Fractional Second"=w2619, "Unix Time (s)"=w2616) -> ("Timestamp"=w2607:timestamp)  [unwired: 8 in, 1 out]
                  n1071 = Format Date/Time String(seconds (now)=w2607, UTC format=TRUE) -> (date/time string=w2608:string)  [unwired: 1 in]
                  n1072 = Scan From String(format string="%<%x %H:%M:%S%3u>T", input string=w2608) -> (output 1=w2609:timestamp)  [unwired: 3 in, 3 out]
                  n1073 = To Double Precision Float(number=w2609) -> (double precision float=w2606:dbl)
                }
                n1074 = Build Path(base path=w2576, name or relative path="Logfile") -> (appended path=w2577:path)
                n1075 = call <vilib>:"Check if File or Folder Exists.vi"("path"=w2577) -> ("file or folder exists?"=w2578:bool, "dup path"=w2579:path)  [unwired: 8 in, 1 out]
                n1076 = case shown="False" w2578 {
                  tunnel: w2579 -> [w2604 w2605]
                  tunnel: [w2603 w2605] -> w2580
                  frame False {
                    n1077 = Create Folder(path (use dialog)=w2604) -> (created path=w2603:path)  [unwired: 2 in, 2 out]
                  }
                  frame True {
                  }
                }
                n1078 = Build Path(base path=w2580, name or relative path=w2583) -> (appended path=w2581:path)
                n1079 = Open/Create/Replace File(file path (use dialog)=w2581, operation (0:open)=T11."open or create") -> (refnum out=w2574:refnum<file>, error out=w2572:errorcluster)  [unwired: 4 in, 1 out]
                n1080 = Write to Text File(file (use dialog)=w2574, text=w2575, error in=w2572) -> (refnum out=w2573:refnum<file>, error out=w2571:errorcluster)  [unwired: 1 in, 1 out]
                n1081 = Close File(refnum=w2573, error in=w2571) -> (path=w2560:path)  [unwired: 1 out]
              }
            }
            "Enabled channels" <- w441
            "CH_Z Graph" <- w453
            "CH_X Graph" <- w452
            "CH_Y Graph" <- w451
            "INC_X Graph" <- w450
            "INC_Y Graph" <- w449
            "File path" <- w444
            n1082 = property on="INC_Y Graph" class="WFChart (strict)"("XScale.Offset"=w443) -> ()  [unwired: 2 in, 2 out]
            n1083 = property on="CH_Z Graph" class="WFChart (strict)"("XScale.Offset"=w448) -> ()  [unwired: 2 in, 2 out]
            n1084 = property on="CH_X Graph" class="WFChart (strict)"("XScale.Offset"=w447) -> ()  [unwired: 2 in, 2 out]
            n1085 = property on="INC_X Graph" class="WFChart (strict)"("XScale.Offset"=w445) -> ()  [unwired: 2 in, 2 out]
            n1086 = property on="CH_Y Graph" class="WFChart (strict)"("XScale.Offset"=w446) -> ()  [unwired: 2 in, 2 out]
            n1087 = call-poly <vilib>:"Write Delimited Spreadsheet.vi"("file path (dialog if empty)"=w444, "format (%s)"="%s", "2D data"=w410, "append to file? (new file:F)"=TRUE, "transpose? (no:F)"=FALSE, "delimiter (\\t)"=";" ("delimiter (\\t)")) -> ()  [unwired: 8 in, 2 out]
          }
          frame 4 {
            w2705 = i16 -1 ("Numeric")
            w2715 = i16 -1 ("Numeric")
            w2721 = i16 -1 ("Numeric")
            # "Determine sign"
            # "Keep only 16 bits"
            # "this block contain measures+ time stamp which saved in the logfile"
            # "this block contain measured values"
            # "this block contain different device type"
            # "function to write headers of the logfile"
            # "function to calculate timestamp"
            n1088 = String Subset(string=w2731, offset (0)=0, length (rest)=16 ("length (rest)")) -> (substring=w2730:string)
            n1089 = String To Byte Array(string=w2819) -> (unsigned byte array=w2829:u8[])
            n1090 = Array Size(array=w2829) -> (size(s)=w2830:i32)
            n1091 = Array To Cluster(array=w2829) -> (cluster=w2838:T15)
            n1092 = Array Subset(array=w2829, index=10, length=4) -> (w2865:u8[])
            n1093 = Array Subset(array=w2829, index=14, length=22) -> (w2860:u8[])
            n1094 = Unbundle(w2838) -> ("unsigned byte array[0]"=w2796:u8, "unsigned byte array[1]"=w2837:u8)
            n1095 = Array To Cluster(array=w2865) -> (cluster=w2864:T12)
            n1096 = Array To Cluster(array=w2860) -> (cluster=w2859:T17)
